vi "Keithley6221_IConstRead.vi"(7 "error in (no error)":errorcluster, 10 "GPIB ADR":u16) -> (0 "error out":errorcluster, 2 "Reading":dbl)   [LabVIEW 2011]
panel:
  out "VISA Refnum out":refnum<visa-resource-name>
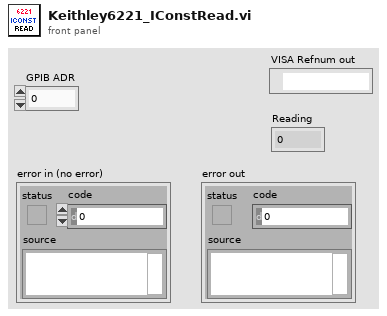
[diagram p1: front panel]
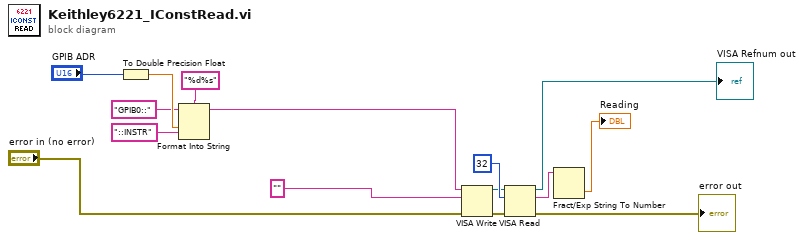
[diagram p0: block diagram]
diagram:
  n1 = To Double Precision Float(number="GPIB ADR") -> (double precision float=w7:dbl)
  n2 = Format Into String(format string="%d%s" ("Removes all labels from the string"), initial string="GPIB0::", w7, "::INSTR") -> (resulting string=w2:string)  [unwired: 1 in, 1 out]
  n3 = VISA Write(VISA resource name=w2, write buffer="", error in (no error)="error in (no error)") -> (VISA resource name out=w9:refnum<visa-resource-name>, error out=w11:errorcluster)  [unwired: 1 out]
  n4 = VISA Read(VISA resource name=w9, byte count=u32 32, error in (no error)=w11) -> (VISA resource name out=→"VISA Refnum out":refnum<visa-resource-name>, read buffer=w14:string, error out=→"error out":errorcluster)  [unwired: 1 out]
  n5 = Fract/Exp String To Number(string=w14) -> (number=→"Reading":dbl)  [unwired: 3 in, 1 out]
